vi "FindOwningLibrary.vi"(10 "Parent":refnum<vi>) -> (2 "Owner":refnum<vi>)   [LabVIEW 2019, in "TestSuite.lvclass"]
uses:
  TestSuite.lvclass
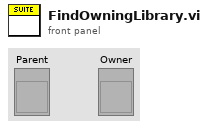
[diagram p1: front panel]
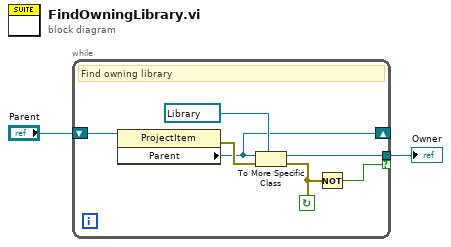
[diagram p0: block diagram]
diagram:
  n1 = while {
    shift-right: [w6] -> _
    shift-left: "Parent" -> [w9]
    tunnel: [w5] -> w1 if=w3
    stop <- w4 continue-if-true
    # "Find owning library"
    n2 = property class="ProjectItem"(reference=w9) -> (error out=w8:errorcluster, "Parent"=w6:refnum<vi>)  [unwired: 1 in, 1 out]
    n3 = To More Specific Class(target class=refnum<vi> refnum ("reference out"), reference=w6, error in=w8) -> (specific class reference=w5:refnum<vi>, error out=w4:errorcluster)
    n4 = Not(x=w4) -> (.not. x?=w3:bool)
  }
  "Owner" <- w1
